vi "Handbetrieb-04-02-17.vi"(4 "AnzahlHorst":i32, 5 "AnzahlHorst/Modul":i32[](array[numeric]), 6 "AnzahlLH":i32, 7 "AnzahlDIOs/Modul":i32[](array[numeric]), 8 "AnzahlDIOs":i32, 9 "Zwangsbedingungen":dbl[][](array[numeric]), 10 "Methodennummer":i32(ring) items=["0"]) -> (1 "Methodennummer":i32(ring) items=["0"])   [LabVIEW 2010]
uses:
  GVMWHorst.vi
  GVZwangs.vi
  GVHK1Hz.vi
  gvbooleschRT.vi
  GVZeitenZyklen.vi
  GVVentilposition.vi
  GVMetavariablen.vi
  GVZwangsMPV.vi
  GVZwangsMPVPos.vi
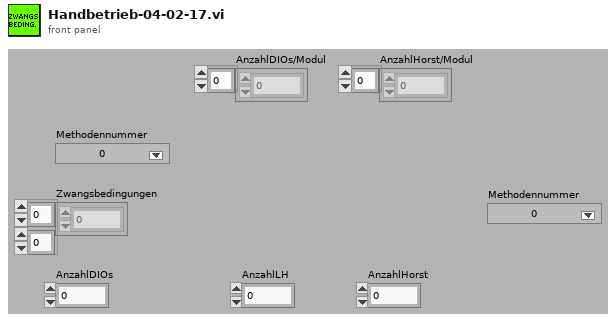
[diagram p1: front panel]
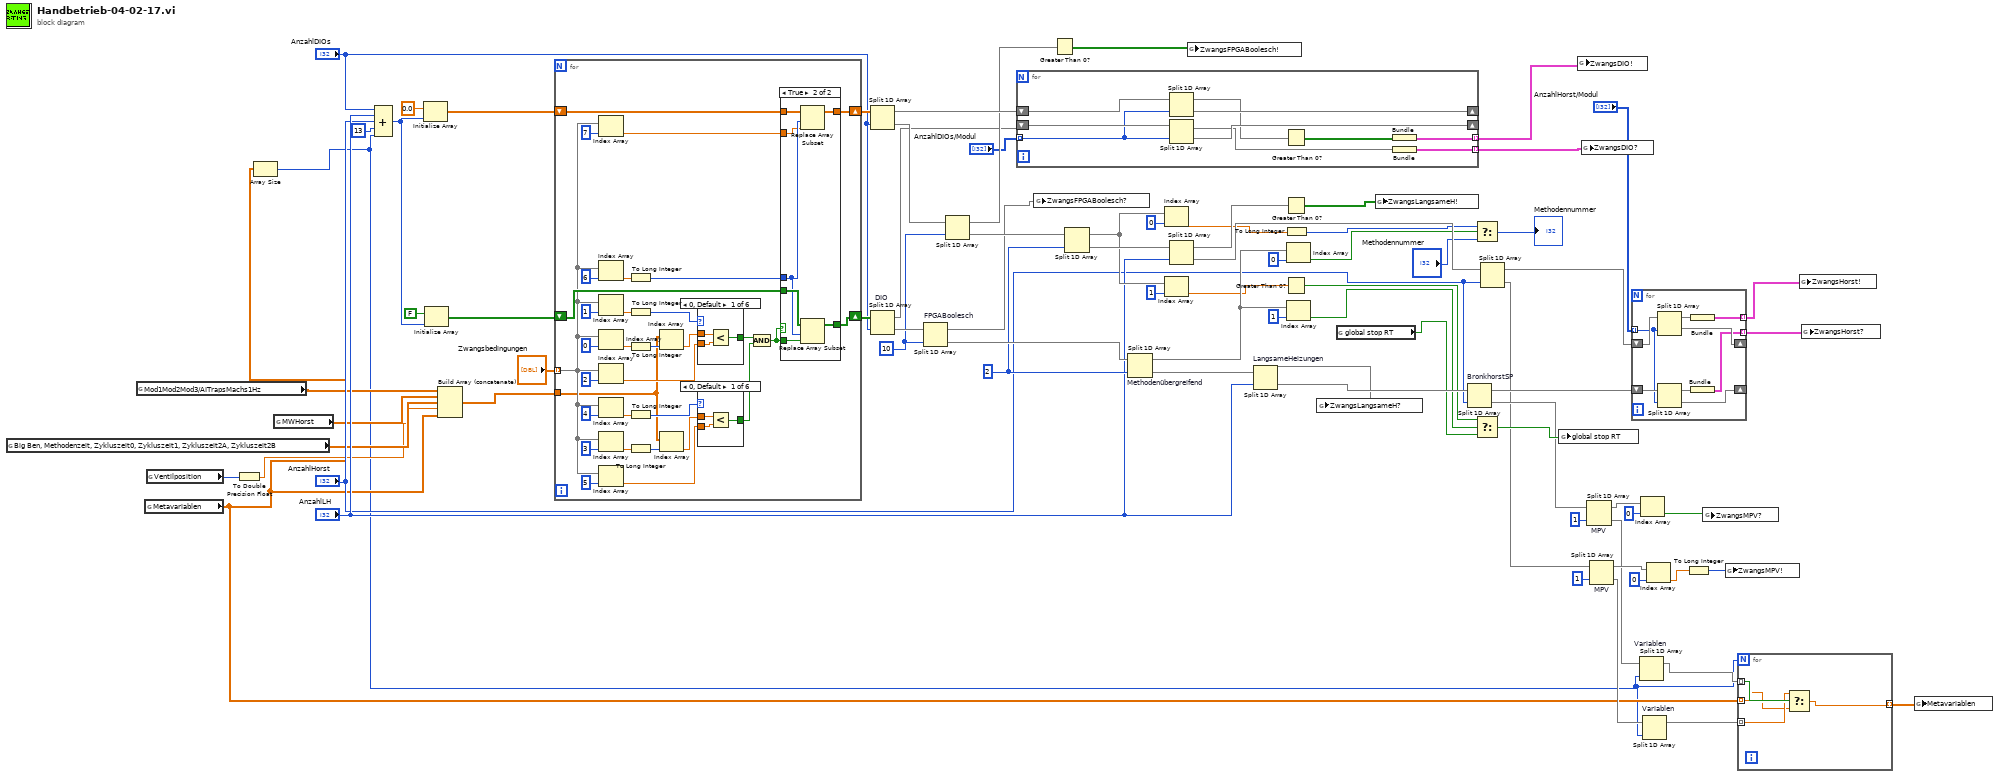
[diagram p0: block diagram]
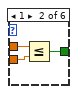
[diagram p2: hidden frame]
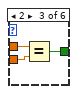
[diagram p3: hidden frame]
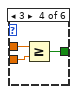
[diagram p4: hidden frame]
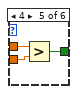
[diagram p5: hidden frame]
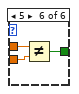
[diagram p6: hidden frame]
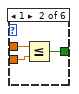
[diagram p8: hidden frame]
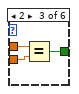
[diagram p9: hidden frame]
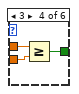
[diagram p10: hidden frame]
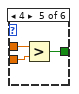
[diagram p11: hidden frame]
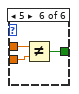
[diagram p12: hidden frame]
diagram:
  w61 = 2 ("Index")
  w71 = 10 ("Index")
  n1 = global read "GVZeitenZyklen.vi" "Big Ben, Methodenzeit, Zykluszeit0, Zykluszeit1, Zykluszeit2A, Zykluszeit2B"() -> (w21:dbl[])
  n2 = global read "GVHK1Hz.vi" "Mod1Mod2Mod3/AITrapsMachs1Hz"() -> (w24:dbl[])
  n3 = global read "GVMetavariablen.vi" "Metavariablen"() -> (w2:dbl[])
  n4 = global read "GVVentilposition.vi" "Ventilposition"() -> (w20:i32)
  n5 = To Double Precision Float(number=w20) -> (double precision float=w19:dbl)
  n6 = Array Size(array=w2) -> (size(s)=w1:i32)
  n7 = global read "GVMWHorst.vi" "MWHorst"() -> (w33:dbl[])
  n8 = Compound Arithmetic op=ADD("AnzahlDIOs", "AnzahlLH", "AnzahlHorst", 13 ("Wert"), w1) -> (w49:i32)
  n9 = Initialize Array(0.0, w49) -> (w46:dbl[])
  n10 = Initialize Array(FALSE, w49) -> (w45:bool[])
  n11 = Build Array (concatenate)(w24, w33, w21, w19, w2) -> (w78:dbl[])
  n12 = for {
    tunnel: w78 -> [w85]
    tunnel: "Zwangsbedingungen" -> [w89] mode=indexing
    shift-right: [w93] -> w77
    shift-left: w45 -> [w98]
    shift-right: [w94] -> w73
    shift-left: w46 -> [w97]
    n13 = Index Array(array=w89, index=7 ("Index")) -> (element=w95:dbl)
    n14 = Index Array(array=w89, index=6 ("Index")) -> (element=w100:dbl)
    n15 = Index Array(array=w89, index=1 ("Index")) -> (element=w107:dbl)
    n16 = Index Array(array=w89, index=0 ("Index")) -> (element=w109:dbl)
    n17 = Index Array(array=w89, index=2 ("Index")) -> (element=w103:dbl)
    n18 = Index Array(array=w89, index=4 ("Index")) -> (element=w83:dbl)
    n19 = Index Array(array=w89, index=3 ("Index")) -> (element=w84:dbl)
    n20 = Index Array(array=w89, index=5 ("Index")) -> (element=w82:dbl)
    n21 = To Long Integer(number=w100) -> (32bit integer=w96:i32)
    n22 = To Long Integer(number=w107) -> (32bit integer=w106:i32)
    n23 = To Long Integer(number=w109) -> (32bit integer=w102:i32)
    n24 = To Long Integer(number=w83) -> (32bit integer=w88:i32)
    n25 = To Long Integer(number=w84) -> (32bit integer=w86:i32)
    n26 = Index Array(array=w85, index=w102) -> (element=w105:dbl)
    n27 = Index Array(array=w85, index=w86) -> (element=w87:dbl)
    n28 = case shown="0, Default" w106 {
      tunnel: w105 -> [w140 w142 w146 w149 w152 w155]
      tunnel: w103 -> [w139 w143 w145 w148 w151 w154]
      tunnel: [w138 w141 w144 w147 w150 w153] -> w80
      frame 0, Default {
        n29 = Less?(x=w140, y=w139) -> (x < y?=w138:bool)
      }
      frame 1 {
        n30 = Less Or Equal?(x=w142, y=w143) -> (x <= y?=w141:bool)
      }
      frame 2 {
        n31 = Equal?(x=w146, y=w145) -> (x = y?=w144:bool)
      }
      frame 3 {
        n32 = Greater Or Equal?(x=w149, y=w148) -> (x >= y?=w147:bool)
      }
      frame 4 {
        n33 = Greater?(x=w152, y=w151) -> (0:w150:bool)
      }
      frame 5 {
        n34 = Not Equal?(x=w155, y=w154) -> (x != y?=w153:bool)
      }
    }
    n35 = case shown="0, Default" w88 {
      tunnel: w87 -> [w113 w115 w119 w122 w125 w128]
      tunnel: w82 -> [w112 w116 w118 w121 w124 w127]
      tunnel: [w111 w114 w117 w120 w123 w126] -> w81
      frame 0, Default {
        n36 = Less?(x=w113, y=w112) -> (x < y?=w111:bool)
      }
      frame 1 {
        n37 = Less Or Equal?(x=w115, y=w116) -> (x <= y?=w114:bool)
      }
      frame 2 {
        n38 = Equal?(x=w119, y=w118) -> (x = y?=w117:bool)
      }
      frame 3 {
        n39 = Greater Or Equal?(x=w122, y=w121) -> (x >= y?=w120:bool)
      }
      frame 4 {
        n40 = Greater?(x=w125, y=w124) -> (0:w123:bool)
      }
      frame 5 {
        n41 = Not Equal?(x=w128, y=w127) -> (x != y?=w126:bool)
      }
    }
    n42 = And(x=w80, y=w81) -> (x .and. y?=w79:bool)
    n43 = case shown="True" w79 {
      tunnel: w98 -> [w130 w137]
      tunnel: w97 -> [w129 w136]
      tunnel: w96 -> [_ w135]
      tunnel: w79 -> [_ w134]
      tunnel: w95 -> [_ w133]
      tunnel: [w129 w132] -> w94
      tunnel: [w130 w131] -> w93
      frame False {
      }
      frame True {
        n44 = Replace Array Subset(array=w136, new element=w133, index=w135) -> (w132:dbl[])
        n45 = Replace Array Subset(array=w137, new element=w134, index=w135) -> (w131:bool[])
      }
    }
  }
  n46 = Split 1D Array ("DIO")(array=w73, index="AnzahlDIOs") -> (first subarray=w72:dbl[], second subarray=w70:dbl[])
  n47 = Split 1D Array "DIO"(array=w77, index="AnzahlDIOs") -> (first subarray=w56:bool[], second subarray=w76:bool[])
  n48 = Split 1D Array "FPGABoolesch"(array=w76, index=w71) -> (first subarray=w32:bool[], second subarray=w65:bool[])
  n49 = Split 1D Array(array=w70, index=w71) -> (first subarray=w69:dbl[], second subarray=w63:dbl[])
  n50 = for {
    tunnel: [w158] -> w27 mode=indexing
    tunnel: "AnzahlDIOs/Modul" -> [w160] mode=indexing
    tunnel: [w156] -> w28 mode=indexing
    shift-right: [w164] -> _
    shift-left: w56 -> [w165]
    shift-right: [w162] -> _
    shift-left: w72 -> [w163]
    n51 = Split 1D Array(array=w163, index=w160) -> (first subarray=w161:dbl[], second subarray=w162:dbl[])
    n52 = Split 1D Array(array=w165, index=w160) -> (first subarray=w159:bool[], second subarray=w164:bool[])
    n53 = Greater Than 0?(x=w161) -> (x > 0?=w157:bool[])
    n54 = Bundle(w157) -> (w156:cluster{bool[]})  [unwired: 1 in]
    n55 = Bundle(w159) -> (w158:cluster{bool[]})  [unwired: 1 in]
  }
  n56 = global write "GVZwangs.vi" "ZwangsFPGABoolesch?"(w32) -> ()
  n57 = Greater Than 0?(x=w69) -> (x > 0?=w31:bool[])
  n58 = Split 1D Array(array=w63, index=w61) -> (first subarray=w57:dbl[], second subarray=w62:dbl[])
  n59 = Split 1D Array "Methodenübergreifend"(array=w65, index=w61) -> (first subarray=w59:bool[], second subarray=w64:bool[])
  n60 = Index Array(array=w57, index=0 ("Index")) -> (element=w38:dbl)
  n61 = Index Array(array=w57, index=1 ("Index")) -> (element=w42:dbl)
  n62 = Split 1D Array(array=w62, index="AnzahlLH") -> (first subarray=w66:dbl[], second subarray=w68:dbl[])
  n63 = global write "GVZwangs.vi" "ZwangsFPGABoolesch!"(w31) -> ()
  n64 = Split 1D Array "LangsameHeizungen"(array=w64, index="AnzahlLH") -> (first subarray=w30:bool[], second subarray=w75:bool[])
  n65 = Greater Than 0?(x=w66) -> (x > 0?=w29:bool[])
  n66 = To Long Integer(number=w38) -> (32bit integer=w36:i32)
  n67 = Greater Than 0?(x=w42) -> (x > 0?=w40:bool)
  n68 = Index Array(array=w59, index=0 ("Index")) -> (element=w37:bool)
  n69 = Index Array(array=w59, index=1 ("Index")) -> (element=w41:bool)
  n70 = global write "GVZwangs.vi" "ZwangsLangsameH?"(w30) -> ()
  n71 = global read "gvbooleschRT.vi" "global stop RT"() -> (w23:bool)
  n72 = global write "GVZwangs.vi" "ZwangsLangsameH!"(w29) -> ()
  n73 = Split 1D Array "BronkhorstSP"(array=w75, index="AnzahlHorst") -> (first subarray=w74:bool[], second subarray=w18:bool[])
  n74 = Select(t=w36, s=w37, f="Methodennummer") -> (s? t:f=→"Methodennummer":i32)
  n75 = Select(t=w40, s=w41, f=w23) -> (s? t:f=w22:bool)
  n76 = Split 1D Array(array=w68, index="AnzahlHorst") -> (first subarray=w67:dbl[], second subarray=w15:dbl[])
  n77 = global write "gvbooleschRT.vi" "global stop RT"(w22) -> ()
  n78 = global write "GVZwangs.vi" "ZwangsDIO!"(w28) -> ()
  n79 = global write "GVZwangs.vi" "ZwangsDIO?"(w27) -> ()
  n80 = Split 1D Array "MPV"(array=w18, index=1 ("Index")) -> (first subarray=w14:bool[], second subarray=w7:bool[])
  n81 = Split 1D Array "MPV"(array=w15, index=1 ("Index")) -> (first subarray=w10:dbl[], second subarray=w6:dbl[])
  n82 = for {
    tunnel: "AnzahlHorst/Modul" -> [w171] mode=indexing
    shift-right: [w173] -> _
    shift-left: w74 -> [w174]
    tunnel: [w168] -> w25 mode=indexing
    shift-right: [w170] -> _
    shift-left: w67 -> [w172]
    tunnel: [w166] -> w26 mode=indexing
    n83 = Split 1D Array(array=w172, index=w171) -> (first subarray=w167:dbl[], second subarray=w170:dbl[])
    n84 = Split 1D Array(array=w174, index=w171) -> (first subarray=w169:bool[], second subarray=w173:bool[])
    n85 = Bundle(w167) -> (w166:cluster{dbl[]})  [unwired: 1 in]
    n86 = Bundle(w169) -> (w168:cluster{bool[]})  [unwired: 1 in]
  }
  n87 = Split 1D Array "Variablen"(array=w7, index=w1) -> (first subarray=w5:bool[])  [unwired: 1 out]
  n88 = Index Array(array=w14, index=0 ("Index")) -> (element=w12:bool)
  n89 = Split 1D Array "Variablen"(array=w6, index=w1) -> (first subarray=w4:dbl[])  [unwired: 1 out]
  n90 = Index Array(array=w10, index=0 ("Index")) -> (element=w9:dbl)
  n91 = To Long Integer(number=w9) -> (32bit integer=w8:i32)
  n92 = global write "GVZwangsMPV.vi" "ZwangsMPV?"(w12) -> ()
  n93 = global write "GVZwangsMPVPos.vi" "ZwangsMPV!"(w8) -> ()
  n94 = for {
    N: w1 -> [_]
    tunnel: w5 -> [w178] mode=indexing
    tunnel: w4 -> [w177] mode=indexing
    tunnel: w2 -> [w176] mode=indexing
    tunnel: [w175] -> w3 mode=indexing
    n95 = Select(t=w177, s=w178, f=w176) -> (s? t:f=w175:dbl)
  }
  n96 = global write "GVZwangs.vi" "ZwangsHorst!"(w26) -> ()
  n97 = global write "GVZwangs.vi" "ZwangsHorst?"(w25) -> ()
  n98 = global write "GVMetavariablen.vi" "Metavariablen"(w3) -> ()
